vi "Set Progress Max.vi"(8 "error in (no error)":errorcluster {"code" format="Error %.0f"}, 10 "Progress Max":i32, 11 "UI Interaction in":refnum<class "UI Interaction.lvclass">) -> (0 "error out":errorcluster {"code" format="Error %.0f"}, 3 "UI Interaction out":refnum<class "UI Interaction.lvclass">)   [LabVIEW 2023, in "UI Interaction.lvclass"]
doc: "Sets the Progress Max, which is can be used to set the max value on a progress bar or the like."
uses:
  UI Interaction.lvclass
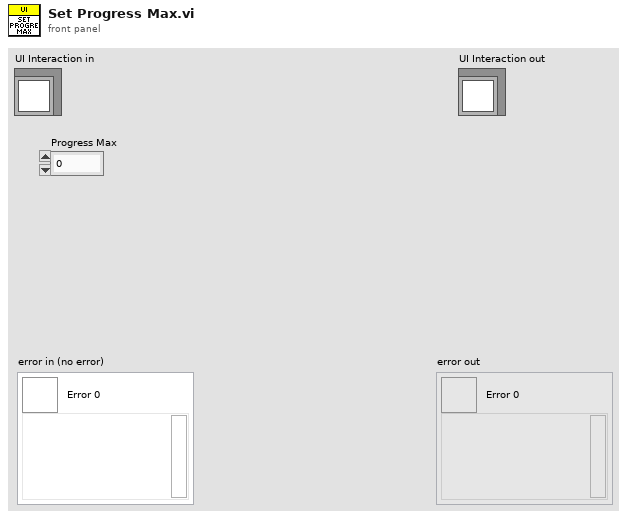
[diagram p1: front panel]
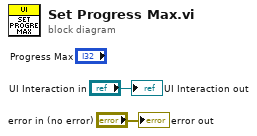
[diagram p0: block diagram]
diagram:
  "error out" <- "error in (no error)"
  "UI Interaction out" <- "UI Interaction in"
